vi "FindColllisionPoints.vi"(6 "enemy_robots":T1[](array[typedef]), 7 "our_robots":T1[](array[typedef]), 8 "Robot in":T1, 9 "Goal":dbl[](array[numeric]), 10 "Initial State":dbl[](array[numeric]), 11 "ball":dbl[](array[numeric])) -> (2 "Collision Points":dbl[][](array[numeric]))   [LabVIEW 2018]
uses:
  Core/AI Robot.ctl
  Intel/Functions Enum.ctl
  Intel/AttackerStates.ctl
  PathDests.ctl
  PathDest.ctl
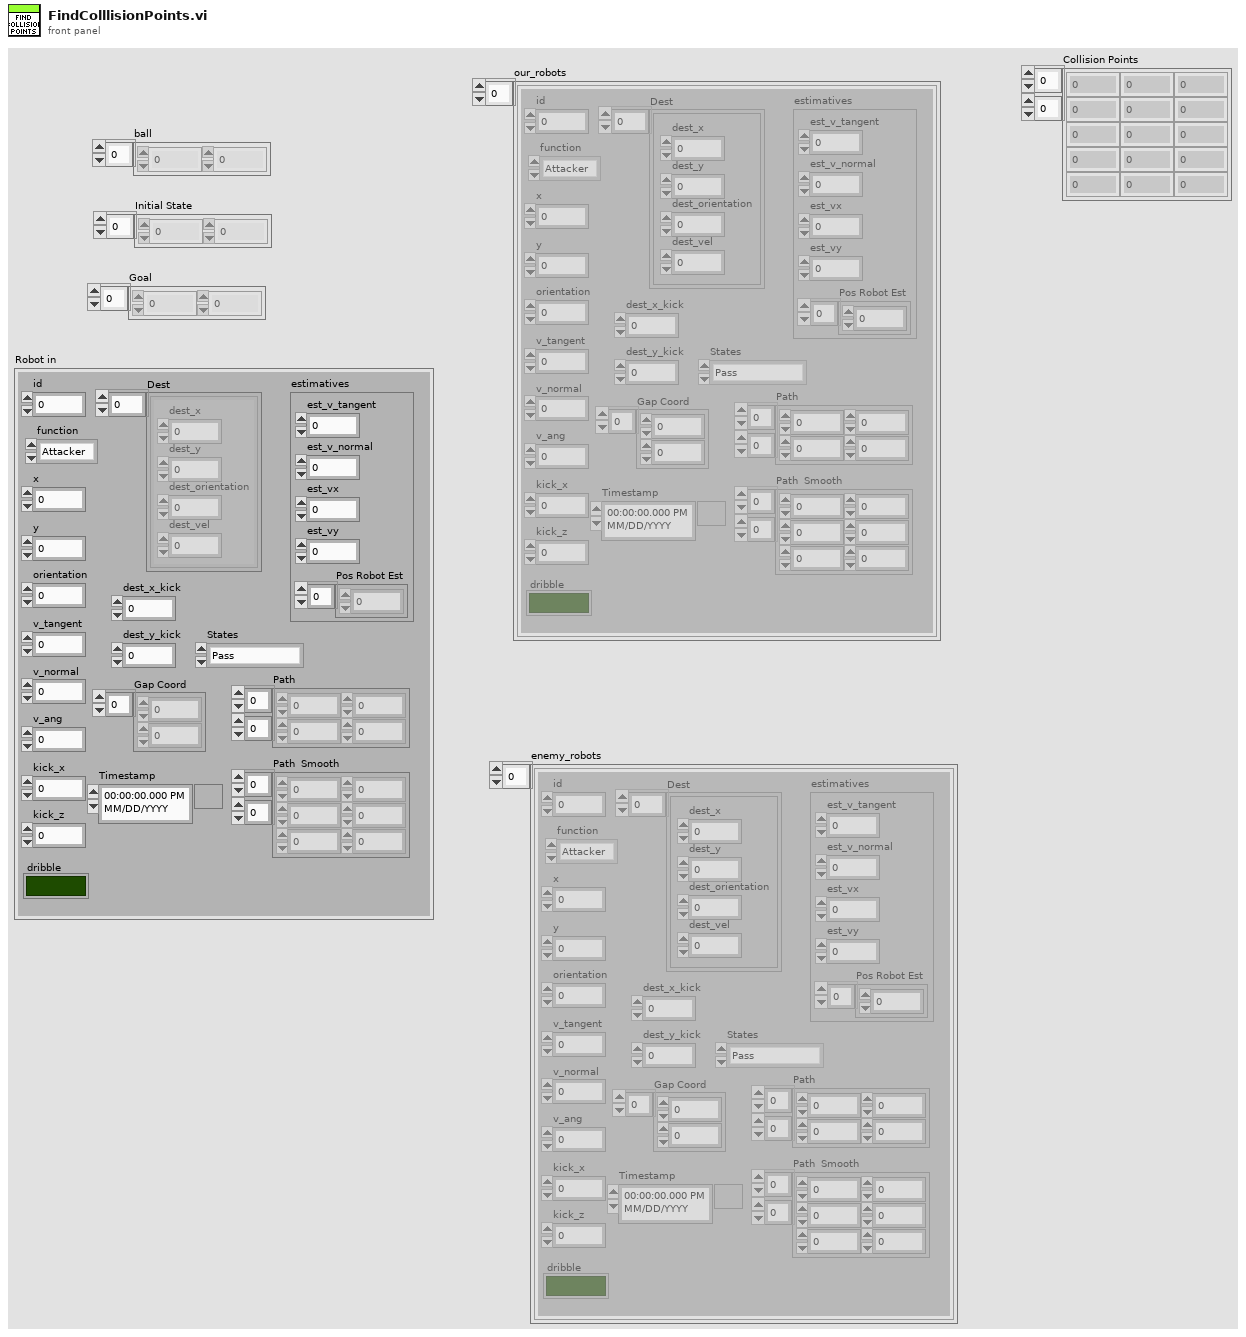
[diagram p1: front panel]
types:
  T1 = typedef "AI Robot.ctl" = cluster{"id":u32, "function":T2, "x":dbl, "y":dbl, "orientation":dbl, "v_tangent":dbl, "v_normal":dbl, "v_ang":dbl, "kick_x":dbl, "kick_z":dbl, "dribble":bool, "Timestamp":timestamp, "estimatives":cluster{"est_v_tangent":dbl, "est_v_normal":dbl, "est_vx":dbl, "est_vy":dbl, "Pos Robot Est":dbl[]}, "dest_x_kick":dbl, "dest_y_kick":dbl, "Gap Coord":dbl[], "States":T3, "Path ":dbl[][], "Path  Smooth":dbl[][], "Dest":T4}
  T2 = typedef "Functions Enum.ctl" = enum16{"Attacker", "Goalie", "Defender", "Striker", "Goto 0", "Dummy", "Kicker", "ZigZag"}
  T3 = typedef "AttackerStates.ctl" = enum16{"Pass", "GoToTangent", "BallGetting", "GoToKick", "Rotate anti-clockwise", "Rotate Clockwise", ""}
  T4 = typedef "PathDests.ctl" = T5[]
  T5 = typedef "PathDest.ctl" = cluster{"dest_x":dbl, "dest_y":dbl, "dest_orientation":dbl, "dest_vel":dbl}
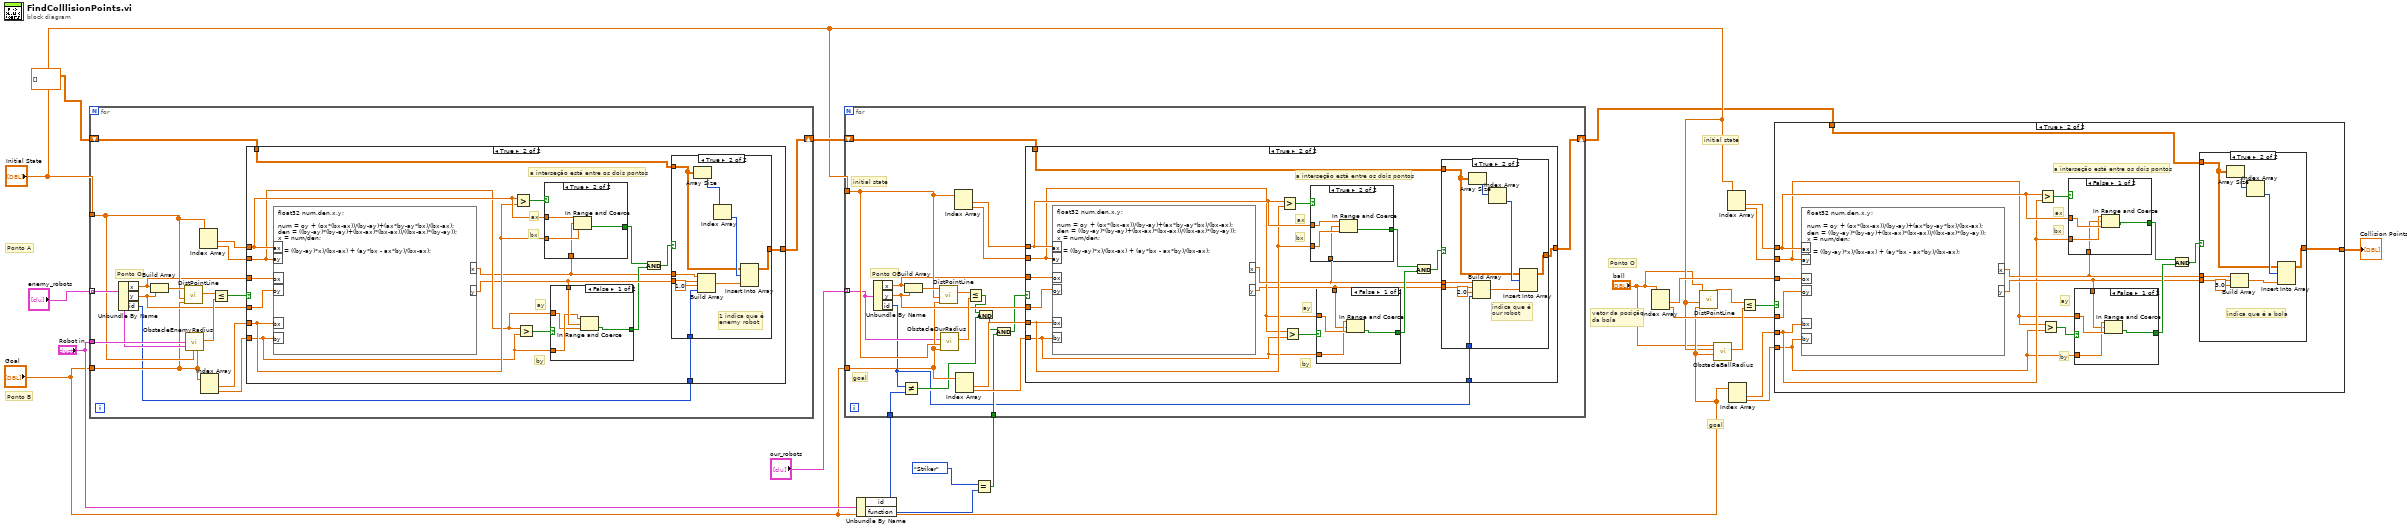
[diagram p0: block diagram]
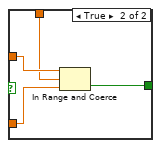
[diagram p4: hidden frame]
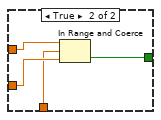
[diagram p5: hidden frame]
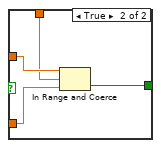
[diagram p8: hidden frame]
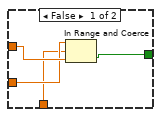
[diagram p9: hidden frame]
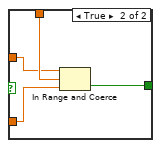
[diagram p12: hidden frame]
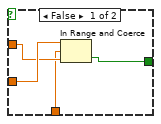
[diagram p13: hidden frame]
diagram:
  # "goal"
  # "initial state"
  # "Ponto O"
  # "vetor da posição\nda bola"
  # "Ponto B"
  # "Ponto A"
  n1 = for {
    tunnel: "enemy_robots" -> [w36] mode=indexing
    tunnel: "Initial State" -> [w32]
    tunnel: "Goal" -> [w27]
    tunnel: "Robot in" -> [w37]
    shift-right: [w33] -> w21
    shift-left: dbl[][] [] ("Path") -> [w34]
    # "Ponto O"
    n2 = Unbundle By Name(w36) -> ("x"=w29:dbl, "y"=w28:dbl, "id"=w24:u32)
    n3 = Build Array(w29, w28) -> (w40:dbl[])
    n4 = call "DistPointLine.vi"("P2"=w27, "P1"=w32, "Q"=w40) -> ("distance"=w39:dbl)  [unwired: 8 in]
    n5 = call "ObstacleEnemyRadius.vi"("Goal"=w27, "Initial State"=w32, "Robot enemy"=w36, "Robot in"=w37) -> ("obstacle enemy radius"=w38:dbl)  [unwired: 7 in]
    n6 = Index Array(array=w32) -> (element #1=w31:dbl, element #2=w30:dbl)  [unwired: 2 in]
    n7 = Index Array(array=w27) -> (element #1=w26:dbl, element #2=w25:dbl)  [unwired: 2 in]
    n8 = Less Or Equal?(x=w39, y=w38) -> (x <= y?=w35:bool)
    n9 = case shown="True" w35 {
      tunnel: w34 -> [w41 w55]
      tunnel: [w41 w54] -> w33
      tunnel: w31 -> [_ w52]
      tunnel: w30 -> [_ w49]
      tunnel: w29 -> [_ w57]
      tunnel: w28 -> [_ w56]
      tunnel: w26 -> [_ w51]
      tunnel: w25 -> [_ w48]
      tunnel: w24 -> [_ w42]
      frame False {
        # "obstáculo longe da trajetória"
      }
      frame True {
        # "a interseção está entre os dois pontos"
        # "by"
        # "ay"
        # "bx"
        # "ax"
        n10 = formula code="float32 num,den,x,y;\n\nnum = oy + (ox*(bx-ax))/(by-ay)+(ax*by-ay*bx)/(bx-ax);\nden = ((by-ay)*(by-ay)+(bx-ax)*(bx-ax))/((bx-ax)*(by-ay));\nx = num/den;\n\ny = ((by-ay)*x)/(bx-ax) + (ay*bx - ax*by)/(bx-ax);"("ax"=w52, "ay"=w49, "ox"=w57, "oy"=w56, "bx"=w51, "by"=w48) -> ("x"=w44:sgl, "y"=w47:sgl)
        n11 = Greater?(x=w52, y=w51) -> (0:w53:bool)
        n12 = Greater?(x=w49, y=w48) -> (0:w50:bool)
        n13 = case shown="True" w53 {
          tunnel: w52 -> [w78 w83]
          tunnel: w51 -> [w79 w82]
          tunnel: [w77 w81] -> w46
          tunnel: w44 -> [w76 w80]
          frame False {
            n14 = In Range and Coerce(upper limit=w79, x=w76, lower limit=w78) -> (In Range?=w77:bool)  [unwired: 1 out]
          }
          frame True {
            n15 = In Range and Coerce(upper limit=w83, x=w80, lower limit=w82) -> (In Range?=w81:bool)  [unwired: 1 out]
          }
        }
        n16 = case shown="False" w50 {
          tunnel: [w71 w75] -> w45
          tunnel: w49 -> [w68 w73]
          tunnel: w48 -> [w69 w72]
          tunnel: w47 -> [w70 w74]
          frame False {
            n17 = In Range and Coerce(upper limit=w69, x=w70, lower limit=w68) -> (In Range?=w71:bool)  [unwired: 1 out]
          }
          frame True {
            n18 = In Range and Coerce(upper limit=w73, x=w74, lower limit=w72) -> (In Range?=w75:bool)  [unwired: 1 out]
          }
        }
        n19 = And(x=w46, y=w45) -> (x .and. y?=w43:bool)
        n20 = case shown="True" w43 {
          tunnel: w55 -> [w58 w64]
          tunnel: [w58 w63] -> w54
          tunnel: w47 -> [_ w62]
          tunnel: w44 -> [_ w61]
          tunnel: w42 -> [_ w59]
          frame False {
          }
          frame True {
            # "1 indica que é\nenemy robot"
            n21 = Array Size(array=w64) -> (size(s)=w67:i32[])
            n22 = Build Array(w61, w62, sgl 1.0 ("element"), w59) -> (w65:sgl[])
            n23 = Index Array(array=w67) -> (element=w66:i32)  [unwired: 1 in]
            n24 = Insert Into Array(array=w64, index (row)=w66, new element=w65) -> (w63:dbl[][])  [unwired: 1 in]
          }
        }
      }
    }
  }
  n25 = Unbundle By Name("Robot in") -> ("id"=w18:u32, "function"=w3:T2)
  n26 = Equal?(x=Functions_Enum."Striker", y=w3) -> (x = y?=w1:bool)
  n27 = for {
    tunnel: "our_robots" -> [w91] mode=indexing
    tunnel: "Initial State" -> [w99]
    tunnel: "Goal" -> [w94]
    shift-right: [w100] -> w5
    shift-left: w21 -> [w101]
    tunnel: w18 -> [w90]
    tunnel: w1 -> [w86]
    # "goal"
    # "initial state"
    # "Ponto O"
    n28 = Unbundle By Name(w91) -> ("x"=w96:dbl, "y"=w95:dbl, "id"=w84:u32)
    n29 = Not Equal?(x=w84, y=w90) -> (x != y?=w88:bool)
    n30 = Build Array(w96, w95) -> (w104:dbl[])
    n31 = call "DistPointLine.vi"("P2"=w94, "P1"=w99, "Q"=w104) -> ("distance"=w103:dbl)  [unwired: 8 in]
    n32 = call "ObstacleOurRadius.vi"("Goal"=w94, "Initial State"=w99, "other robot"=w91) -> ("obstacle enemy radius"=w102:dbl)  [unwired: 8 in]
    n33 = Index Array(array=w99) -> (element #1=w98:dbl, element #2=w97:dbl)  [unwired: 2 in]
    n34 = Index Array(array=w94) -> (element #1=w93:dbl, element #2=w92:dbl)  [unwired: 2 in]
    n35 = Less Or Equal?(x=w103, y=w102) -> (x <= y?=w89:bool)
    n36 = And(x=w89, y=w88) -> (x .and. y?=w87:bool)
    n37 = And(x=w87, y=w86) -> (x .and. y?=w85:bool)
    n38 = case shown="True" w85 {
      tunnel: w101 -> [w105 w119]
      tunnel: [w105 w118] -> w100
      tunnel: w98 -> [_ w113]
      tunnel: w97 -> [_ w110]
      tunnel: w96 -> [_ w121]
      tunnel: w95 -> [_ w120]
      tunnel: w93 -> [_ w112]
      tunnel: w92 -> [_ w109]
      tunnel: w84 -> [_ w106]
      frame False {
        # "obstáculo longe da trajetória"
      }
      frame True {
        # "a interseção está entre os dois pontos"
        # "by"
        # "ay"
        # "bx"
        # "ax"
        n39 = formula code="float32 num,den,x,y;\n\nnum = oy + (ox*(bx-ax))/(by-ay)+(ax*by-ay*bx)/(bx-ax);\nden = ((by-ay)*(by-ay)+(bx-ax)*(bx-ax))/((bx-ax)*(by-ay));\nx = num/den;\n\ny = ((by-ay)*x)/(bx-ax) + (ay*bx - ax*by)/(bx-ax);"("ax"=w113, "ay"=w110, "ox"=w121, "oy"=w120, "bx"=w112, "by"=w109) -> ("x"=w111:sgl, "y"=w108:sgl)
        n40 = Greater?(x=w113, y=w112) -> (0:w117:bool)
        n41 = Greater?(x=w110, y=w109) -> (0:w116:bool)
        n42 = case shown="True" w117 {
          tunnel: [w143 w147] -> w115
          tunnel: w113 -> [w142 w146]
          tunnel: w112 -> [w141 w145]
          tunnel: w111 -> [w140 w144]
          frame False {
            n43 = In Range and Coerce(upper limit=w141, x=w140, lower limit=w142) -> (In Range?=w143:bool)  [unwired: 1 out]
          }
          frame True {
            n44 = In Range and Coerce(upper limit=w146, x=w144, lower limit=w145) -> (In Range?=w147:bool)  [unwired: 1 out]
          }
        }
        n45 = case shown="False" w116 {
          tunnel: [w135 w139] -> w114
          tunnel: w110 -> [w134 w138]
          tunnel: w109 -> [w133 w137]
          tunnel: w108 -> [w132 w136]
          frame False {
            n46 = In Range and Coerce(upper limit=w133, x=w132, lower limit=w134) -> (In Range?=w135:bool)  [unwired: 1 out]
          }
          frame True {
            n47 = In Range and Coerce(upper limit=w138, x=w136, lower limit=w137) -> (In Range?=w139:bool)  [unwired: 1 out]
          }
        }
        n48 = And(x=w115, y=w114) -> (x .and. y?=w107:bool)
        n49 = case shown="True" w107 {
          tunnel: w119 -> [w122 w128]
          tunnel: [w122 w127] -> w118
          tunnel: w111 -> [_ w126]
          tunnel: w108 -> [_ w125]
          tunnel: w106 -> [_ w123]
          frame False {
          }
          frame True {
            # "indica que é \nour robot"
            n50 = Array Size(array=w128) -> (size(s)=w131:i32[])
            n51 = Build Array(w126, w125, sgl 2.0 ("element"), w123) -> (w129:sgl[])
            n52 = Index Array(array=w131) -> (element=w130:i32)  [unwired: 1 in]
            n53 = Insert Into Array(array=w128, index (row)=w130, new element=w129) -> (w127:dbl[][])  [unwired: 1 in]
          }
        }
      }
    }
  }
  n54 = Index Array(array="ball") -> (element #1=w10:dbl, element #2=w9:dbl)  [unwired: 2 in]
  n55 = call "DistPointLine.vi"("P2"="Goal", "P1"="Initial State", "Q"="ball") -> ("distance"=w17:dbl)  [unwired: 8 in]
  n56 = call "ObstacleBallRadius.vi"("Goal"="Goal", "Initial State"="Initial State", "ball"="ball") -> ("obstacle enemy radius"=w16:dbl)  [unwired: 8 in]
  n57 = Index Array(array="Initial State") -> (element #1=w14:dbl, element #2=w13:dbl)  [unwired: 2 in]
  n58 = Index Array(array="Goal") -> (element #1=w12:dbl, element #2=w11:dbl)  [unwired: 2 in]
  n59 = Less Or Equal?(x=w17, y=w16) -> (x <= y?=w15:bool)
  n60 = case shown="True" w15 {
    tunnel: [w148 w153] -> w4
    tunnel: w14 -> [_ w152]
    tunnel: w13 -> [_ w149]
    tunnel: w10 -> [_ w163]
    tunnel: w9 -> [_ w162]
    tunnel: w12 -> [_ w151]
    tunnel: w11 -> [_ w150]
    tunnel: w5 -> [w148 w154]
    frame False {
      # "obstáculo longe da trajetória"
    }
    frame True {
      # "a interseção está entre os dois pontos"
      # "by"
      # "ay"
      # "bx"
      # "ax"
      n61 = formula code="float32 num,den,x,y;\n\nnum = oy + (ox*(bx-ax))/(by-ay)+(ax*by-ay*bx)/(bx-ax);\nden = ((by-ay)*(by-ay)+(bx-ax)*(bx-ax))/((bx-ax)*(by-ay));\nx = num/den;\n\ny = ((by-ay)*x)/(bx-ax) + (ay*bx - ax*by)/(bx-ax);"("ax"=w152, "ay"=w149, "ox"=w163, "oy"=w162, "bx"=w151, "by"=w150) -> ("x"=w156:sgl, "y"=w155:sgl)
      n62 = Greater?(x=w152, y=w151) -> (0:w161:bool)
      n63 = Greater?(x=w149, y=w150) -> (0:w160:bool)
      n64 = case shown="False" w161 {
        tunnel: [w184 w188] -> w159
        tunnel: w152 -> [w183 w187]
        tunnel: w151 -> [w182 w186]
        tunnel: w156 -> [w181 w185]
        frame False {
          n65 = In Range and Coerce(upper limit=w182, x=w181, lower limit=w183) -> (In Range?=w184:bool)  [unwired: 1 out]
        }
        frame True {
          n66 = In Range and Coerce(upper limit=w187, x=w185, lower limit=w186) -> (In Range?=w188:bool)  [unwired: 1 out]
        }
      }
      n67 = case shown="False" w160 {
        tunnel: [w176 w180] -> w158
        tunnel: w149 -> [w175 w179]
        tunnel: w150 -> [w174 w178]
        tunnel: w155 -> [w173 w177]
        frame False {
          n68 = In Range and Coerce(upper limit=w174, x=w173, lower limit=w175) -> (In Range?=w176:bool)  [unwired: 1 out]
        }
        frame True {
          n69 = In Range and Coerce(upper limit=w179, x=w177, lower limit=w178) -> (In Range?=w180:bool)  [unwired: 1 out]
        }
      }
      n70 = And(x=w159, y=w158) -> (x .and. y?=w157:bool)
      n71 = case shown="True" w157 {
        tunnel: w154 -> [w164 w169]
        tunnel: [w164 w168] -> w153
        tunnel: w156 -> [_ w167]
        tunnel: w155 -> [_ w166]
        frame False {
        }
        frame True {
          # "indica que é a bola"
          n72 = Array Size(array=w169) -> (size(s)=w172:i32[])
          n73 = Build Array(w167, w166, sgl 3.0 ("element")) -> (w170:sgl[])
          n74 = Index Array(array=w172) -> (element=w171:i32)  [unwired: 1 in]
          n75 = Insert Into Array(array=w169, index (row)=w171, new element=w170) -> (w168:dbl[][])  [unwired: 1 in]
        }
      }
    }
  }
  "Collision Points" <- w4
